vi "time生成路径 (子VI).vi"(10 "名称或相对路径":string="ORP滴定曲线\\", 11 "时间":string) -> (3 "appended path":path)   [LabVIEW 2016, in "斯坦道CODMn新电路板.lvlib"]
uses:
  <vilib>/Utility/sysdir.llb/System Directory Type.ctl
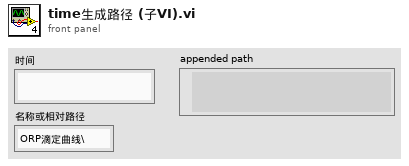
[diagram p1: front panel]
types:
  T1 = typedef "System Directory Type.ctl" = i32
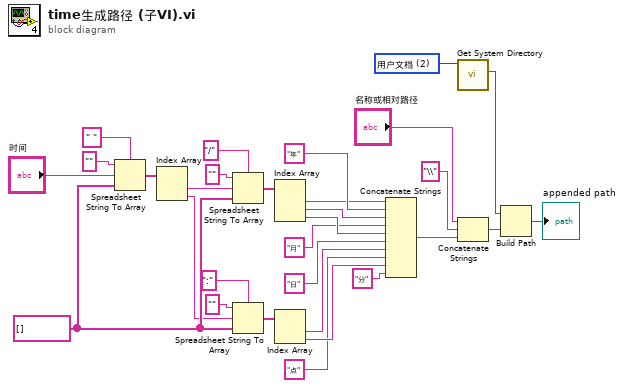
[diagram p0: block diagram]
diagram:
  w26 = T1 2 items=["用户目录"=0, "用户桌面"=1, "用户文档"=2, "用户应用程序数据"=3, "用户设置"=4, "用户临时目录"=5, "公共文档"=6, "公共应用程序数据"=7, "公共设置"=8, "公共缓存"=13, "系统核心库"=9, "系统安装库"=10, "应用程序文件"=11, "启动盘根目录"=12] ("system directory type")
  w20 = string[] []
  n1 = Spreadsheet String To Array(delimiter (Tab)=" " ("分隔符(Tab)"), format string="" ("格式字符串"), spreadsheet string="时间", array type (2D Dbl)=w20) -> (array=w4:string[])
  n2 = Index Array(array=w4) -> (element #1=w9:string, element #2=w19:string)  [unwired: 2 in]
  n3 = Spreadsheet String To Array(delimiter (Tab)="/" ("分隔符(Tab)"), format string="" ("格式字符串"), spreadsheet string=w9, array type (2D Dbl)=w20) -> (array=w10:string[])
  n4 = Spreadsheet String To Array(delimiter (Tab)=":" ("分隔符(Tab)"), format string="" ("格式字符串"), spreadsheet string=w19, array type (2D Dbl)=w20) -> (array=w21:string[])
  n5 = Index Array(array=w10) -> (element #1=w11:string, element #2=w13:string, element #3=w15:string)  [unwired: 3 in]
  n6 = Index Array(array=w21) -> (element #1=w22:string, element #2=w24:string)  [unwired: 2 in]
  n7 = Concatenate Strings(w11, "年" ("替换字符串(\"\")"), w13, "月" ("替换字符串(\"\")"), w15, "日" ("替换字符串(\"\")"), w22, "点" ("替换字符串(\"\")"), w24, "分" ("字符串")) -> (w29:string)
  n8 = call <vilib>:"Get System Directory.vi"("system directory type"=w26) -> ("system directory"=w27:path)  [unwired: 10 in]
  n9 = Concatenate Strings("名称或相对路径", "\\" ("名称或相对路径"), w29) -> (w28:string)
  n10 = Build Path(base path=w27, name or relative path=w28) -> (appended path=→"appended path":path)
